vi "Valve Picture.vi"(7 "Valve Pictures":T2, 10 "Unused Element":T1, 11 "Values":T7) -> (2 "Valve Picture":picture)   [LabVIEW 2020, in "VolatusGUIElements.lvlib" / "2WayValveV.lvclass"]
uses:
  2WayValveV.lvclass
  Values.ctl
  Channel State.ctl
  Valve Pictures.ctl
  Command Pictures.ctl
  Picture.ctl
  Feedback Pictures.ctl
  Energized Pictures.ctl
  Unused Element.ctl
  Picture.vi
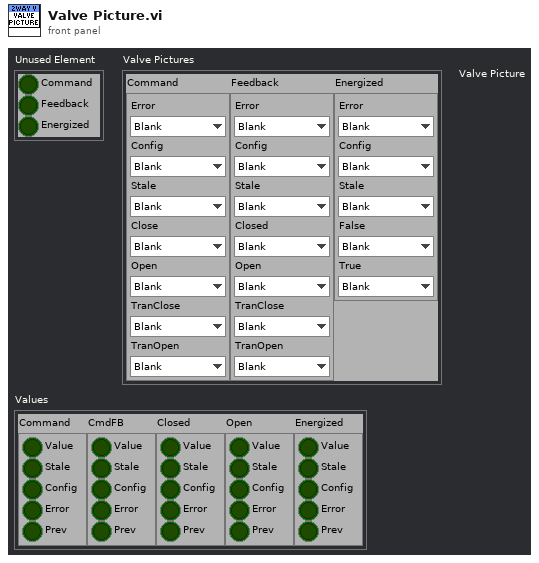
[diagram p1: front panel]
types:
  T1 = typedef "VolatusGUIElements.lvlib/2WayValveV.lvclass/Unused Element.ctl" = cluster{"Command":bool, "Feedback":bool, "Energized":bool}
  T2 = typedef "VolatusGUIElements.lvlib/2WayValveV.lvclass/Valve Pictures.ctl" = cluster{"Command":T3, "Feedback":T5, "Energized":T6}
  T3 = typedef "VolatusGUIElements.lvlib/2WayValveV.lvclass/Command Pictures.ctl" = cluster{"Error":T4, "Config":T4, "Stale":T4, "Close":T4, "Open":T4, "TranClose":T4, "TranOpen":T4}
  T4 = typedef "VolatusGUIElements.lvlib/2WayValveV.lvclass/Picture.ctl" = enum16{"Blank", "OutClose", "OutOpen", "OutTranClose", "OutTranOpen", "OutConfig", "OutStale", "OutError", "InClose", "InOpen", "InTranClose", "InTranOpen", "InConfig", "InStale", "InError", "EnOff", "EnOn", "EnConfig", "EnStale", "EnError"}
  T5 = typedef "VolatusGUIElements.lvlib/2WayValveV.lvclass/Feedback Pictures.ctl" = cluster{"Error":T4, "Config":T4, "Stale":T4, "Closed":T4, "Open":T4, "TranClose":T4, "TranOpen":T4}
  T6 = typedef "VolatusGUIElements.lvlib/2WayValveV.lvclass/Energized Pictures.ctl" = cluster{"Error":T4, "Config":T4, "Stale":T4, "False":T4, "True":T4}
  T7 = typedef "VolatusGUIElements.lvlib/2WayValveV.lvclass/Values.ctl" = cluster{"Command":T8, "CmdFB":T8, "Closed":T8, "Open":T8, "Energized":T8}
  T8 = typedef "VolatusGUIElements.lvlib/2WayValveV.lvclass/Channel State.ctl" = cluster{"Value":bool, "Stale":bool, "Config":bool, "Error":bool, "Prev":bool}
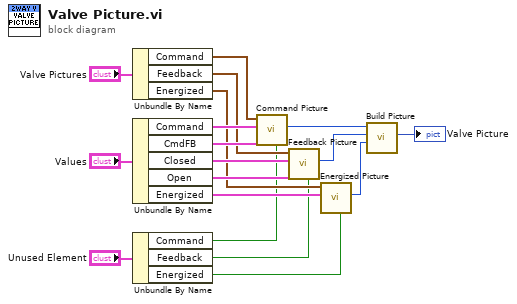
[diagram p0: block diagram]
diagram:
  n1 = Unbundle By Name("Valve Pictures") -> ("Command"=w16:T3, "Feedback"=w12:T5, "Energized"=w9:T6)
  n2 = Unbundle By Name("Values") -> ("Command"=w15:T8, "CmdFB"=w14:T8, "Closed"=w13:T8, "Open"=w11:T8, "Energized"=w10:T8)
  n3 = Unbundle By Name("Unused Element") -> ("Command"=w5:bool, "Feedback"=w6:bool, "Energized"=w7:bool)
  n4 = call "Command Picture.vi"("Unused"=w5, "Feedback State"=w14, "Command State"=w15, "Command Pictures"=w16) -> ("Command Picture"=w4:T4)  [unwired: 7 in]
  n5 = call "Feedback Picture.vi"("Unused"=w6, "Open State"=w11, "Closed State"=w13, "Feedback Pictures"=w12) -> ("Feedback Picture"=w3:T4)  [unwired: 7 in]
  n6 = call "Energized Picture.vi"("Unused"=w7, "Energized State"=w10, "Energized Pictures"=w9) -> ("Energized Picture"=w2:T4)  [unwired: 8 in]
  n7 = call "Build Picture.vi"("Energized Picture"=w2, "Feedback Picture"=w3, "Command Picture"=w4) -> ("Valve Picture"=→"Valve Picture":picture)  [unwired: 8 in]
